vi "PH_Powermeter_BaseClass.PC set Connection.vi"(0 "VI in":refnum<vi>, 2 "Connection":T1, 5 "error in (no error)":errorcluster) -> (14 "VI out":refnum<vi>, 19 "error out":errorcluster)   [LabVIEW 2014, in "PH_Powermeter_BaseClass.lvlib"]
uses:
  PH_Powermeter_BaseClass.lvlib
  PH_Powermeter_BaseClass.Connection.ctl
  PH_Powermeter_BaseClass.State.ctl
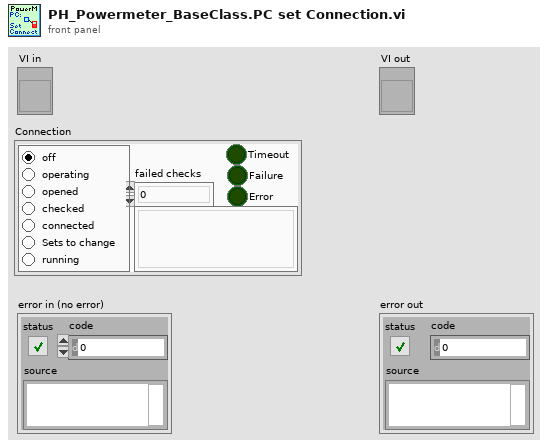
[diagram p1: front panel]
types:
  T1 = typedef "PH_Powermeter_BaseClass.lvlib/PH_Powermeter_BaseClass.Connection.ctl" = cluster{"failed checks":i8, "Timeout":bool, "Data read":string, "Failure":bool, "Error":bool, "State":T2}
  T2 = typedef "PH_Powermeter_BaseClass.lvlib/PH_Powermeter_BaseClass.State.ctl" = enum32{"off", "operating", "opened", "checked", "connected", "Sets to change", "running"}
  T3 = typedef "PH_Powermeter_BaseClass.lvlib/PH_Powermeter_BaseClass.i attribute.ctl" = cluster{"GUI References":T4, "Connection":T1, "Head Attributes":T5, "VISA resource":refnum<visa-resource-name>, "Energy":T6, "Service ID Energy":i32, "Wanted Settings":T7, "Current Settings":T7}
  T4 = typedef "PH_Powermeter_BaseClass.lvlib/PH_Powermeter_BaseClass.GUI Refs.ctl" = cluster{"Head Attributes":refnum<vi>, "Energy":refnum<vi>, "Connection":refnum<vi>, "VISA Resource":refnum<vi>, "Energy evolution":refnum<vi>, "Scaling Factor":refnum<vi>, "Range":refnum<vi>, "Wavelength":refnum<vi>, "Trigger Level":refnum<vi>, "Wanted Settings":refnum<vi>, "Current Settings":refnum<vi>}
  T5 = typedef "PH_Powermeter_BaseClass.lvlib/PH_Powermeter_BaseClass.Head Attributes.ctl" = cluster{"Instrument Type":string, "Head Version":string, "Head Name":string, "Serial Number":string, "Firmware":string, "Sensor Type":string, "MinimumRange":u32, "Maximum Range":u32, "Min Wavelength":i32, "Max Wavelength":i32}
  T6 = typedef "PH_Powermeter_BaseClass.lvlib/PH_Powermeter_BaseClass.Energy.ctl" = cluster{"current Value":dbl, "unscaled":dbl, "Scaling Factor":dbl}
  T7 = typedef "PH_Powermeter_BaseClass.lvlib/PH_gentec_BaseClass.Head Settings.ctl" = cluster{"Trigger Level":dbl, "Wavelength":u32, "Range":u32}
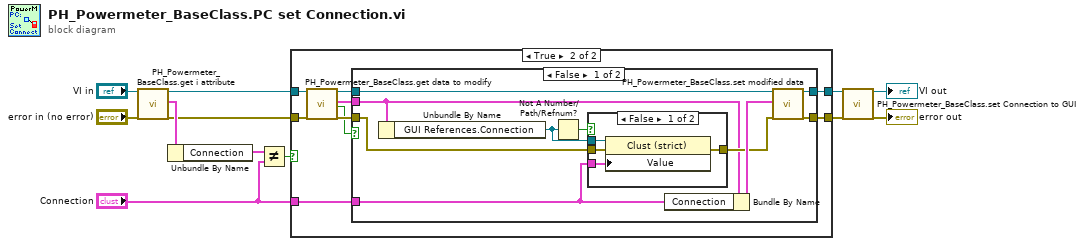
[diagram p0: block diagram]
diagram:
  n1 = call "PH_Powermeter_BaseClass.get i attribute.vi"("i ref in"="VI in", "error in (no error)"="error in (no error)") -> ("i ref out"=w5:refnum<vi>, "i attribute"=w7:T3, "error out"=w6:errorcluster)  [unwired: 15 in]
  n2 = Unbundle By Name(w7) -> ("Connection"=w8:T1)
  n3 = Not Equal?(x=w8, y="Connection") -> (x != y?=w9:bool)
  n4 = case shown="True" w9 {
    tunnel: w5 -> [w14 w19]
    tunnel: w6 -> [w13 w18]
    tunnel: "Connection" -> [_ w17]
    tunnel: [w14 w16] -> w1
    tunnel: [w13 w15] -> w3
    frame False {
    }
    frame True {
      n5 = call "PH_Powermeter_BaseClass.get data to modify.vi"("i ref in"=w19, "error in (no error)"=w18) -> ("i ref out"=w23:refnum<vi>, "i attribute"=w21:T3, "timed out"=w20:bool, "error out"=w22:errorcluster)  [unwired: 14 in]
      n6 = case shown="False" w20 {
        tunnel: [w33 w40] -> w16
        tunnel: [w32 w39] -> w15
        tunnel: w22 -> [w29 w39]
        tunnel: w23 -> [w31 w40]
        tunnel: w21 -> [w27 _]
        tunnel: w17 -> [w24 _]
        frame False {
          n7 = Unbundle By Name(w27) -> ("GUI References.Connection"=w25:refnum<vi>)
          n8 = Not A Number/Path/Refnum?(number/path/refnum=w25) -> (NaN/Path/Refnum?=w26:bool)
          n9 = case shown="False" w26 {
            tunnel: w29 -> [w37 w38]
            tunnel: [w36 w38] -> w28
            tunnel: w25 -> [w35 _]
            tunnel: w24 -> [w34 _]
            frame False {
              n10 = property class="Clust (strict)"(reference=w35, error in=w37, "Value"=w34) -> (error out=w36:errorcluster)  [unwired: 1 out]
            }
            frame True {
            }
          }
          n11 = Bundle By Name(cluster=w27, "Connection"=w24) -> (w30:T3)
          n12 = call "PH_Powermeter_BaseClass.set modified data.vi"("i ref in"=w31, "i attribute"=w30, "error in (no error)"=w28) -> ("i ref out"=w33:refnum<vi>, "error out"=w32:errorcluster)  [unwired: 15 in]
        }
        frame True {
        }
      }
    }
  }
  n13 = call "PH_Powermeter_BaseClass.set Connection to GUI.vi"("i ref in"=w1, "error in"=w3) -> ("i ref out"=→"VI out":refnum<vi>, "error out"=→"error out":errorcluster)  [unwired: 16 in]
